vi "_mallocWithLength.vi"(10 "error in (no error)":errorcluster, 11 "Common.Data Length":i32) -> (2 "error out":errorcluster, 3 "MDPtr DVR":refnum<data-value>)   [LabVIEW 2017, in "MDPtr.lvlib"]
uses:
  MDPtr.lvlib
  MDPtr TypeDef/MDPtr DataFrame-Memory.ctl
  MDPtr TypeDef/MDPtr DataFrame-Common.ctl
  <vilib>/Utility/Data Type/Type Definitions/Data Type.ctl
  <vilib>/Utility/Data Type/NI_Data Type.lvlib
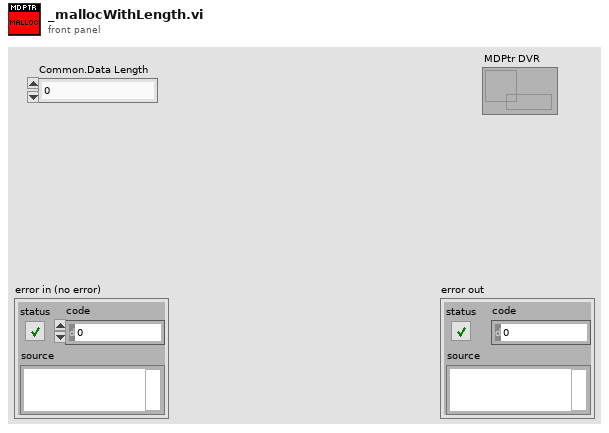
[diagram p1: front panel]
types:
  T1 = typedef "MDPtr.lvlib/MDPtr DataFrame-Memory.ctl" = cluster{"Common":T2, "DVR":refnum<data-value>}
  T2 = typedef "MDPtr.lvlib/MDPtr DataFrame-Common.ctl" = cluster{"Data Type":T3, "Copy Count":i32, "String Attribute":string, "Cache Length":i32, "Data Length":i32}
  T3 = typedef "NI_Data Type.lvlib/Data Type.ctl" = enum8{"Invalid Type", "Void", "I8", "I16", "I32", "I64", "U8", "U16", "U32", "U64", "Single Float", "Double Float", "Extended Float", "Single Complex", "Double Complex", "Extended Complex", "Enum U8", "Enum U16", "Enum U32", "Enum U64", "Single Float With Unit", "Double Float With Unit", "Extended Float With Unit", "Single Complex with Unit", "Double Complex with Unit", "Extended Complex with Unit", "Boolean", "String", "Path", "Picture", "Tag", "Array", "Cluster", "Variant", "LV Variant", "Waveform", "Timestamp", "Digital Waveform", "Digital Data", "ExpressData", "Refnum", "External Data", "VI", "Poly VI", "LabVIEW Class Instance", "Fixed Point"}
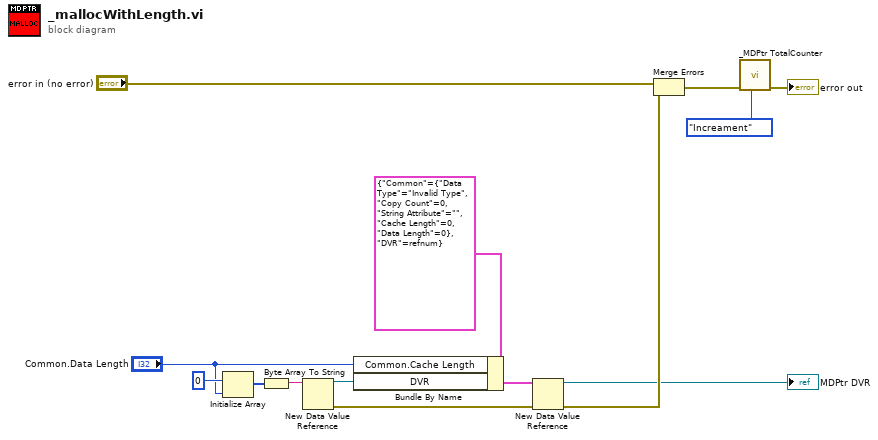
[diagram p0: block diagram]
diagram:
  n1 = Initialize Array(u8 0 ("element"), "Common.Data Length") -> (w2:u8[])
  n2 = Byte Array To String(unsigned byte array=w2) -> (string=w1:string)
  n3 = New Data Value Reference(data value=w1) -> (data value reference=w5:refnum<data-value>, error out=w13:errorcluster)  [unwired: 1 in]
  n4 = Bundle By Name(cluster=T1 {"Common"={"Data Type"=enum."Invalid Type", "Copy Count"=0, "String Attribute"="", "Cache Length"=0, "Data Length"=0}, "DVR"=refnum} ("DataFrame-String"), "Common.Cache Length"="Common.Data Length", "DVR"=w5) -> (w14:T1)
  n5 = New Data Value Reference(data value=w14, error in=w13) -> (data value reference=→"MDPtr DVR":refnum<data-value>, error out=w9:errorcluster)
  n6 = Merge Errors("error in (no error)", w9) -> (w8:errorcluster)
  n7 = call "_MDPtr TotalCounter.vi"("Oper(Get)"=enum16{"GET", "Increament", "decreament"}."Increament", "error in (no error)"=w8) -> ("error out"=→"error out":errorcluster)  [unwired: 8 in, 1 out]
